vi "Overall_system_A0-2_Weightfirst_w_LoadCell.vi"() -> ()   [LabVIEW 2019]
doc: "This VI is th overall VI that can read the weight, rfid and camera (and save the data into a csv file). When certain threshold are met it can also send a telegram message at the end."
uses:
  dependencies/notification/Telegram-Bot-master (1)/Telegram-Bot-master/Telegram/Methods/TypeDefs/SendMessageType.ctl
panel:
  out "Rfid 2":string
  in  "RFID VISA resource name 2":refnum<visa-resource-name>="COM18"
  out "Rfid":string
  in  "RFID VISA resource name":refnum<visa-resource-name>="COM5"
  in  "start rfid (debug)":bool
  out "Weight":string
  in  "delay before read (ms)":u32=500
  in  "Weight VISA resource name":refnum<visa-resource-name>="COM1"
  in  "start condition (debug)":bool
  in  "Start camera (debug)":bool
  out "Health Monitoring in Progress":bool
  in  "Bird is underfeeding (debug)":bool
  out "Current image":T1(plugin-control)
  in  "Camera Name":refnum<k21>="cam0" caption="IMAQdx Session"
  # "Intelligent Health Monitoring System"
  # "grams"
  # "Weight detection settings:"
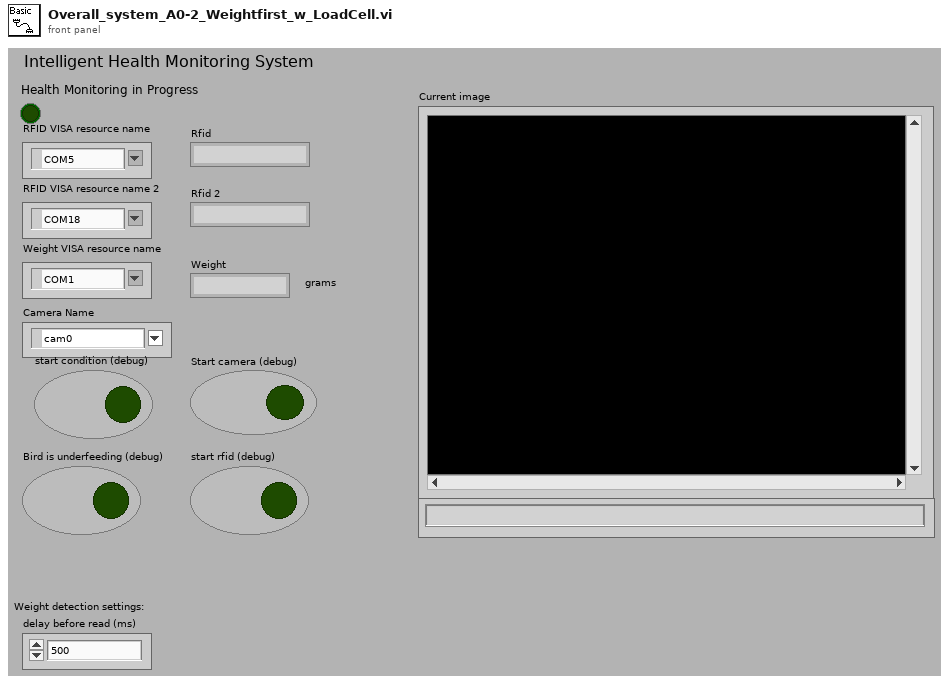
[diagram p1: front panel]
types:
  T1 = typedef "IMAQ Image.ctl" = refnum<image>
  T2 = typedef "SendMessageType.ctl" = enum16{"Text", "ReplyKeyboardMarkup", "ReplyKeyboardRemove"}
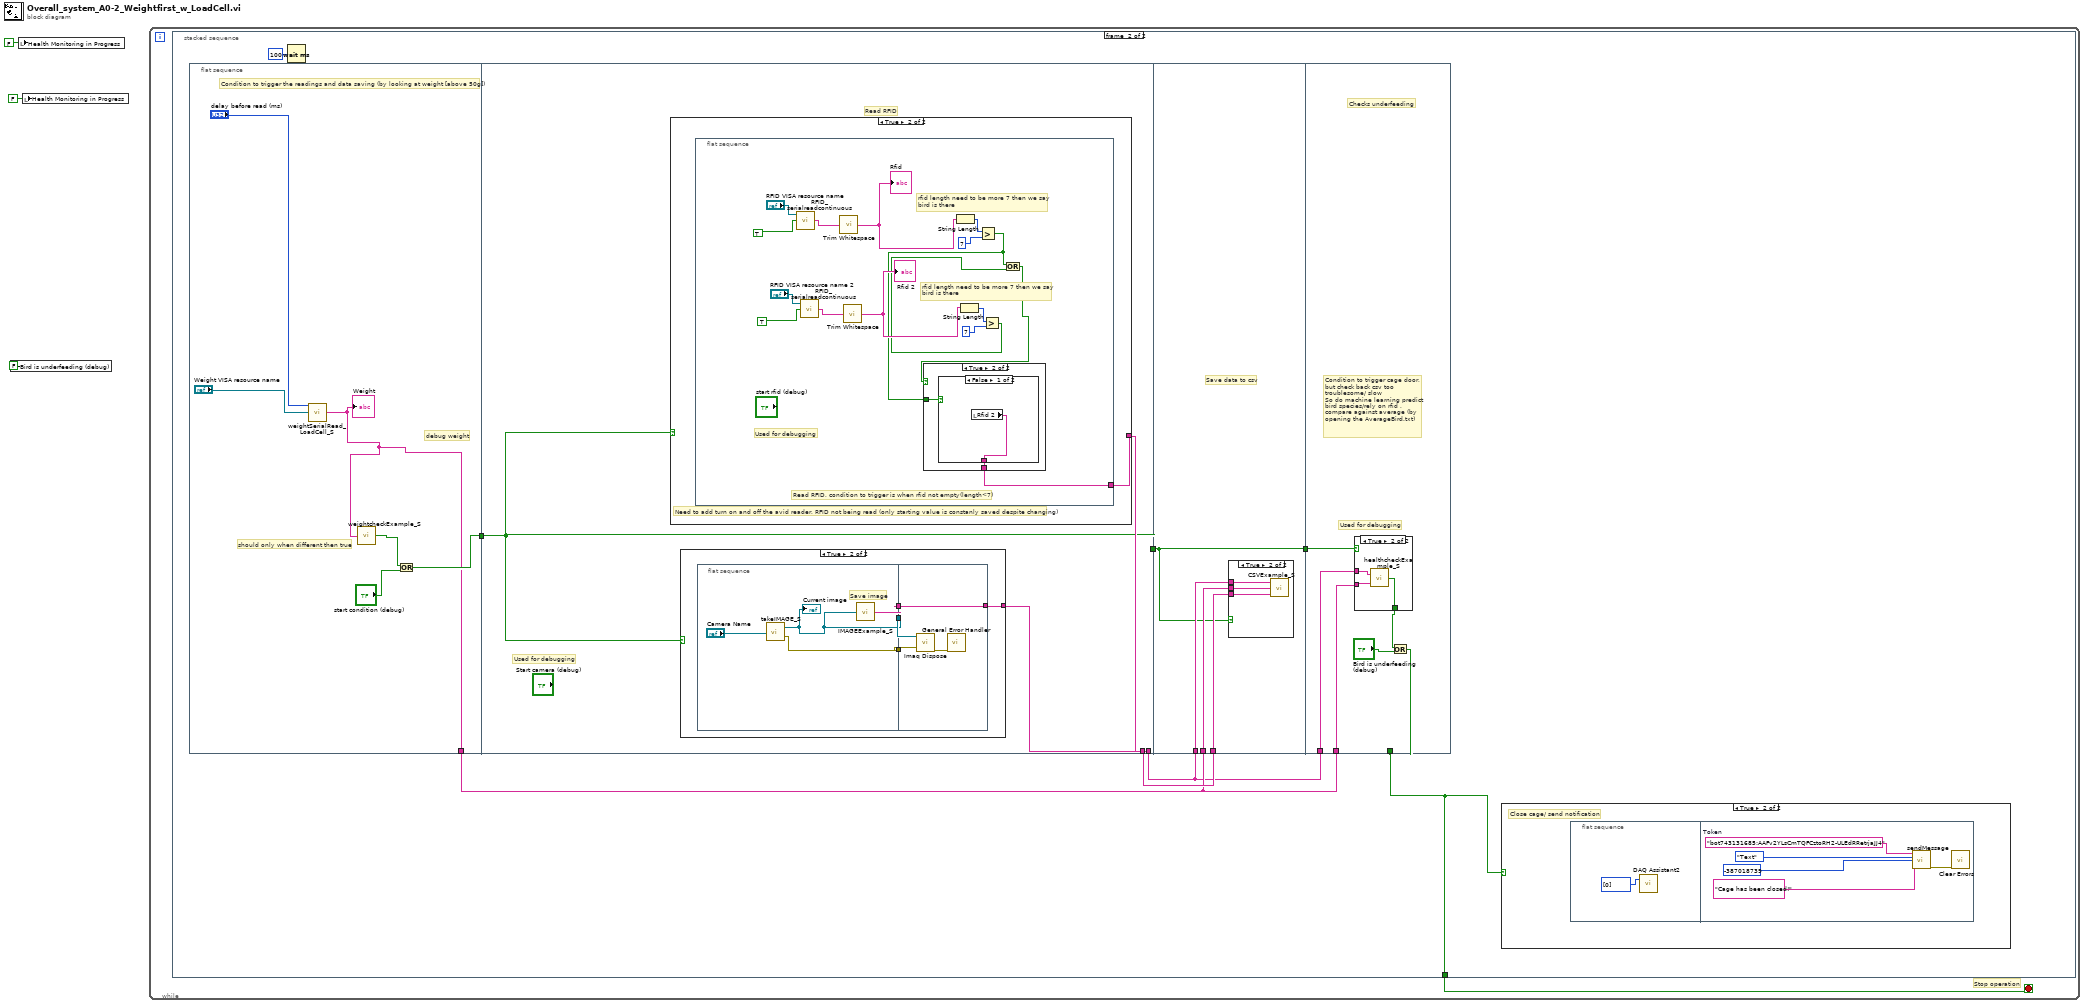
[diagram p0: block diagram]
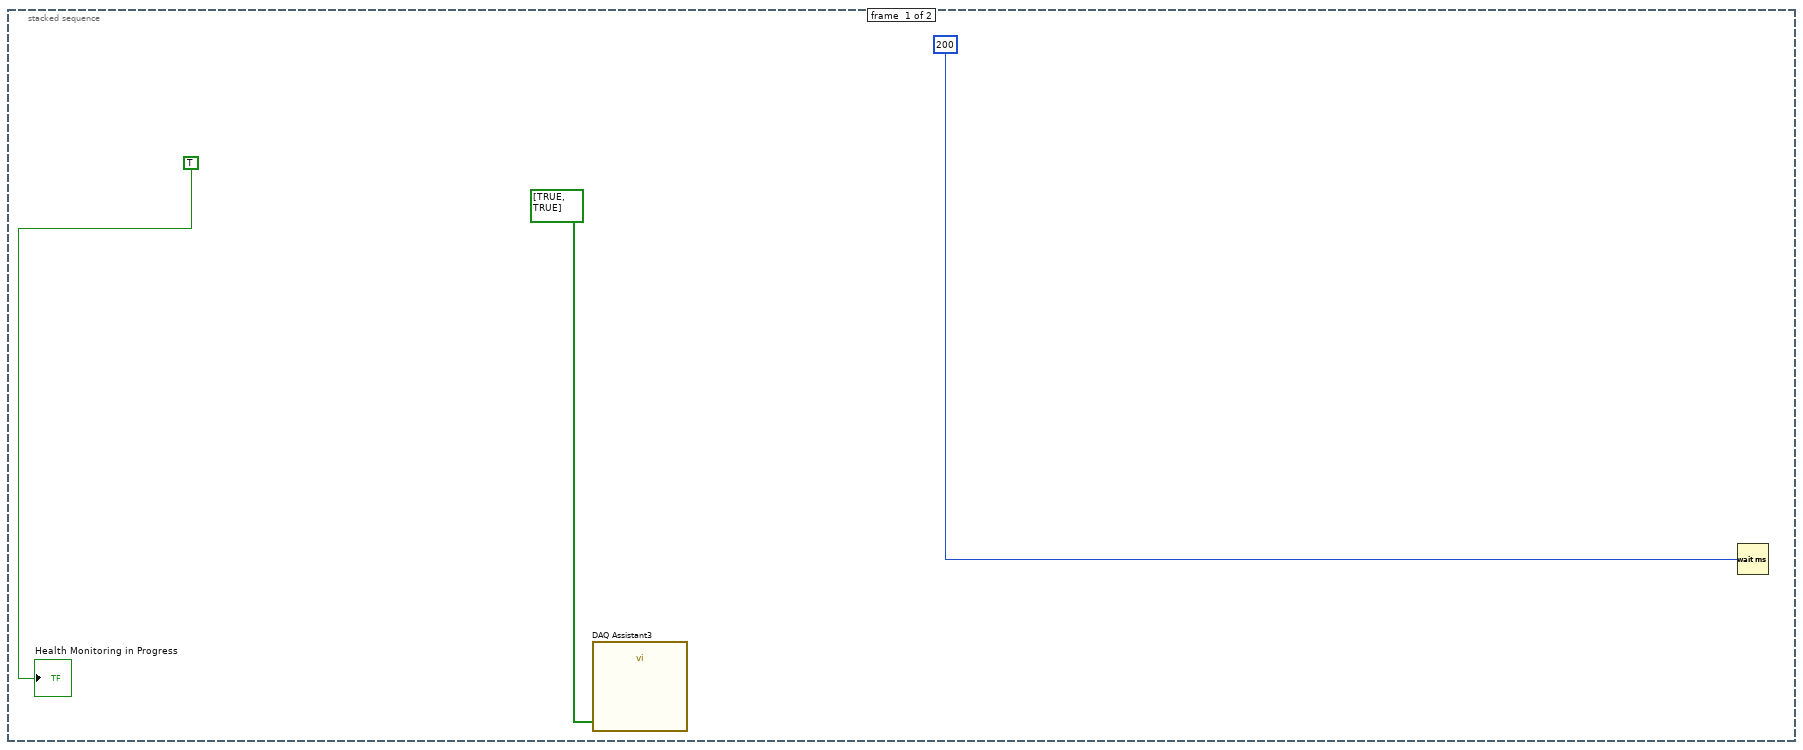
[diagram p2: hidden frame]
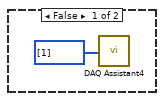
[diagram p4: hidden frame]
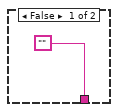
[diagram p5: hidden frame]
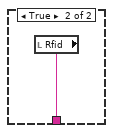
[diagram p6: hidden frame]
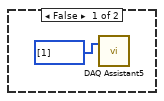
[diagram p9: hidden frame]
diagram:
  n1 = local write "Bird is underfeeding (debug)"(FALSE ("Bird is underfeeding")) -> ()
  n2 = local write "Health Monitoring in Progress"(FALSE ("Health Monitoring in Progress")) -> ()
  n3 = local write "Health Monitoring in Progress"(FALSE ("Health Monitoring in Progress")) -> ()
  n4 = while {
    stop <- w4 stop-if-true
    # "Stop operation"
    n5 = stacked-sequence {
      tunnel: [_ w14] -> w4
      frame #0 {
        n6 = call "DAQ Assistant3"("data"=bool[] [TRUE, TRUE]) -> ()  [unwired: 17 in, 2 out]
        n7 = Wait (ms)(milliseconds to wait=u32 200) -> ()  [unwired: 1 out]
        "Health Monitoring in Progress" <- TRUE ("Health Monitoring in Progress")
      }
      frame #1 {
        n8 = flat-sequence {
          tunnel: [w18] -> w9
          tunnel: [w20] -> w13
          tunnel: [w24] -> w8
          tunnel: [w23] -> w10
          tunnel: w13 -> [w22]
          tunnel: [w22] -> w12
          tunnel: w12 -> [w60]
          tunnel: [w60] -> w11
          tunnel: w10 -> [w63]
          tunnel: w9 -> [w62]
          tunnel: w8 -> [w61]
          tunnel: [w67] -> w14
          tunnel: w9 -> [w72]
          tunnel: w11 -> [w71]
          tunnel: w8 -> [w70]
          frame #0 {
            # "debug weight"
            # "Condition to trigger the readings and data saving (by looking at weight [above 50g])"
            # "should only when different then true"
            n9 = call "weightSerialRead_LoadCell_S.vi"("Weight VISA resource name"="Weight VISA resource name", "delay before read (ms)"="delay before read (ms)") -> ("String"=w18:string)  [unwired: 1 in]
            "Weight" <- w18
            n10 = call "weightcheckExample_S.vi"("weight"=w18) -> ("Boolean"=w19:bool)
            n11 = Or(x=w19, y="start condition (debug)") -> (x .or. y?=w20:bool)
          }
          frame #1 {
            # "Used for debugging"
            # "Read RFID"
            n12 = case shown="True" w22 {
              tunnel: [_ w38] -> w24
              frame False {
                n13 = call "DAQ Assistant4"("data"=u32[] [1]) -> ()  [unwired: 17 in, 2 out]
              }
              frame True {
                # "Need to add turn on and off the avid reader, RFID not being read (only starting value is constanly saved despite changing)"
                n14 = flat-sequence {
                  tunnel: [w39] -> w38
                  frame #0 {
                    # "rfid length need to be more 7 then we say \nbird is there"
                    # "Used for debugging"
                    # "rfid length need to be more 7 then we say \nbird is there"
                    # "Read RFID, condition to trigger is when rfid not empty(length<7)"
                    n15 = call "RFID_serialreadcontinuous.vi"("Read 2"=TRUE, "VISA resource name"="RFID VISA resource name") -> ("Response 2"=w51:string)  [unwired: 1 in]
                    n16 = call "RFID_serialreadcontinuous.vi"("Read 2"=TRUE, "VISA resource name"="RFID VISA resource name 2") -> ("Response 2"=w46:string)  [unwired: 1 in]
                    n17 = call <vilib>:"Trim Whitespace.vi"("string"=w51) -> ("trimmed string"=w52:string)  [unwired: 1 in]
                    "Rfid" <- w52
                    n18 = call <vilib>:"Trim Whitespace.vi"("string"=w46) -> ("trimmed string"=w47:string)  [unwired: 1 in]
                    "Rfid 2" <- w47
                    n19 = String Length(string=w52) -> (length=w54:i32)
                    n20 = String Length(string=w47) -> (length=w48:i32)
                    n21 = Greater?(x=w54, y=7) -> (0:w40:bool)
                    n22 = Greater?(x=w48, y=7) -> (0:w42:bool)
                    n23 = Or(x=w40, y=w42) -> (x .or. y?=w41:bool)
                    n24 = case shown="True" w41 {
                      tunnel: w40 -> [_ w57]
                      tunnel: ["" w56] -> w39
                      frame False {
                      }
                      frame True {
                        n25 = case shown="False" w57 {
                          tunnel: [w58 w59] -> w56
                          frame False {
                            n26 = local read "Rfid 2"() -> (w58:string)
                          }
                          frame True {
                            n27 = local read "Rfid"() -> (w59:string)
                          }
                        }
                      }
                    }
                  }
                }
              }
            }
            n28 = case shown="True" w22 {
              tunnel: [_ w26] -> w23
              frame False {
              }
              frame True {
                n29 = flat-sequence {
                  tunnel: [w30] -> w28
                  tunnel: [w29] -> w27
                  tunnel: [w32] -> w25
                  tunnel: w28 -> [w36]
                  tunnel: w27 -> [w34]
                  tunnel: [w33] -> w26
                  tunnel: w25 -> [w33]
                  frame #0 {
                    # "Save image"
                    n30 = call "takeIMAGE_S.vi"("Camera Name"="Camera Name") -> ("Current image"=w29:T1, "error in (no error)"=w30:errorcluster)
                    "Current image" <- w29
                    n31 = call "IMAGEExample_S.vi"("Image"=w29) -> ("String"=w32:string)
                  }
                  frame #1 {
                    n32 = call "Imaq Dispose"("Image"=w34, "error in (no error)"=w36) -> ("error out"=w35:errorcluster)  [unwired: 4 in]
                    n33 = call <vilib>:"General Error Handler.vi"("error in (no error)"=w35) -> ()  [unwired: 2 in, 13 out]
                  }
                }
              }
            }
          }
          frame #2 {
            # "Save data to csv"
            n34 = case shown="True" w60 {
              tunnel: w63 -> [_ w64]
              tunnel: w62 -> [_ w65]
              tunnel: w61 -> [_ w66]
              frame False {
              }
              frame True {
                n35 = call "CSVExample_S.vi"("imageId"=w64, "weight"=w65, "rfid"=w66) -> ()
              }
            }
          }
          frame #3 {
            # "Used for debugging"
            # "Condition to trigger cage door,\nbut check back csv too troublesome/ slow\nSo do machine learning predict bird species/rely on rfid , compare against average (by opening the AverageBird.txt)"
            # "Checks underfeeding"
            n36 = case shown="True" w71 {
              tunnel: [_ w73] -> w69
              tunnel: w70 -> [_ w74]
              tunnel: w72 -> [_ w75]
              frame False {
              }
              frame True {
                n37 = call "healthcheckExample_S.vi"("weight"=w75, "rfid"=w74) -> ("Boolean"=w73:bool)
              }
            }
            n38 = Or(x=w69, y="Bird is underfeeding (debug)") -> (x .or. y?=w67:bool)
          }
        }
        n39 = Wait (ms)(milliseconds to wait=u32 100) -> ()  [unwired: 1 out]
        n40 = case shown="True" w14 {
          frame False {
            n41 = call "DAQ Assistant5"("data"=u32[] [1]) -> ()  [unwired: 17 in, 2 out]
          }
          frame True {
            # "Close cage/ send notification"
            n42 = flat-sequence {
              frame #0 {
                n43 = call "DAQ Assistant2"("data"=u32[] [0]) -> ()  [unwired: 17 in, 2 out]
              }
              frame #1 {
                w81 = "bot743131685:AAFv2YLsCmTQFCztoRH2-ULEdRRetrjaJJ4"  # Token
                n44 = call "sendMessage.vi"("Token"=w81, "MsgType"=SendMessageType."Text", "ChatId"=i64 -387018739, "Text"="Cage has been closed!") -> ("error out"=w82:errorcluster)  [unwired: 11 in]
                n45 = call <vilib>:"Clear Errors.vi"("error in (no error)"=w82) -> ()  [unwired: 5 in, 2 out]
              }
            }
          }
        }
      }
    }
  }
